vi "array_last_element.vi"(11 "配列":ext[](array[numeric])) -> (3 "最後の要素":ext)   [LabVIEW 2020]
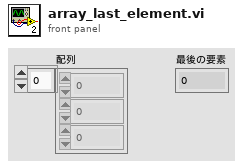
[diagram p1: front panel]
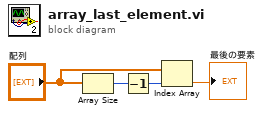
[diagram p0: block diagram]
diagram:
  n1 = Array Size(array="配列") -> (size(s)=w2:i32)
  n2 = Decrement(x=w2) -> (x-1=w3:i32)
  n3 = Index Array(array="配列", index=w3) -> (element=→"最後の要素":ext)
